vi "Draw.vi"(8 "error in (no error)":errorcluster, 10 "2D Picture in":picture, 11 "GrayScaleImage in":refnum<class "GrayScaleImage.lvclass">) -> (0 "error out":errorcluster, 2 "2D Picture out":picture, 3 "GrayScaleImage out":refnum<class "GrayScaleImage.lvclass">)   [LabVIEW 2021, in "Picture2D.lvlib" / "GrayScaleImage.lvclass"]
uses:
  GrayScaleImage.lvclass
  C:/GitHub/Picture2D/src/Picture/Image.lvclass
  ColorGrayScale/ColorGrayScale.lvclass
  Picture/Image.lvclass
  GrayScaleImage.lvclass/GrayScaleImage.ctl
  Picture2D/Picture2D.lvlib
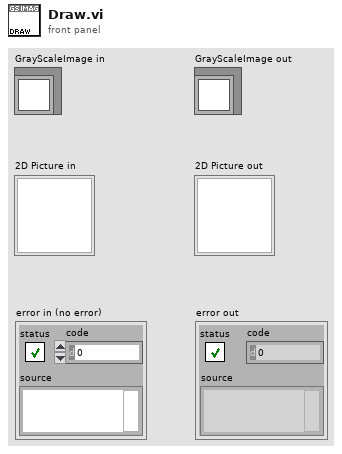
[diagram p1: front panel]
types:
  T1 = typedef "imagedata.ctl" = cluster{"image type":i32, "image depth":i32, "image":u8[], "mask":u8[], "colors":u32[], "Rectangle":cluster{"left":i16, "top":i16, "right":i16, "bottom":i16}}
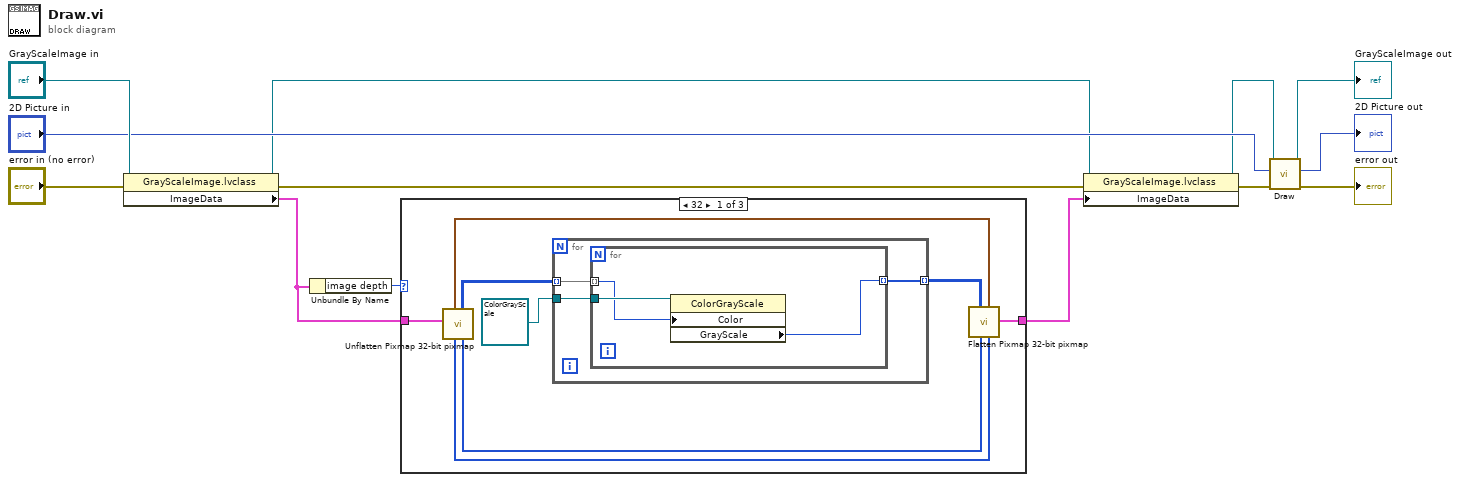
[diagram p0: block diagram]
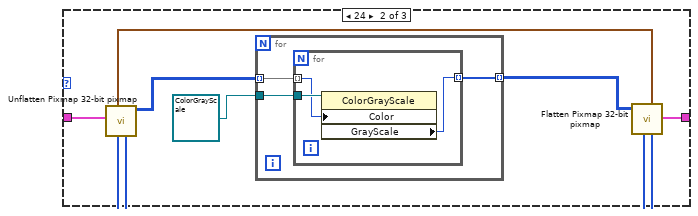
[diagram p2: hidden frame]
diagram:
  n1 = property class="GrayScaleImage.lvclass"(reference="GrayScaleImage in", error in="error in (no error)") -> (reference out=w2:refnum<class "GrayScaleImage.lvclass">, error out=w5:errorcluster, "ImageData"=w10:T1)
  n2 = Unbundle By Name(w10) -> ("image depth"=w13:i32)
  n3 = case shown="32" w13 {
    tunnel: w10 -> [w21 w35 w42]
    tunnel: [w20 w34 w42] -> w3
    frame 32 {
      n4 = call "Unflatten Pixmap 32-bit pixmap.vi"("image data"=w21) -> ("colors"=w17:u32[], "32-bit pixmap"=w15:u32[][], "mask"=w18:u8[], "top left"=w19:cluster{"x":i16, "y":i16})  [unwired: 3 in, 4 out]
      n5 = for {
        tunnel: refnum<class "ColorGrayScale.lvclass"> refnum ("ColorGrayScale") -> [w24]
        tunnel: [w23] -> w14 mode=indexing
        tunnel: w15 -> [w22] mode=indexing
        n6 = for {
          tunnel: w24 -> [w27]
          tunnel: [w25] -> w23 mode=indexing
          tunnel: w22 -> [w26] mode=indexing
          n7 = property class="ColorGrayScale"(reference=w27, "Color"=w26) -> ("GrayScale"=w25:u32)  [unwired: 1 in, 2 out]
        }
      }
      n8 = call "Flatten Pixmap 32-bit pixmap.vi"("mask"=w18, "top left"=w19, "colors"=w17, "32-bit pixmap"=w14) -> ("image data"=w20:T1)  [unwired: 7 in]
    }
    frame 24 {
      n9 = call "Unflatten Pixmap 32-bit pixmap.vi"("image data"=w35) -> ("24-bit pixmap"=w29:u32[][], "colors"=w31:u32[], "mask"=w32:u8[], "top left"=w33:cluster{"x":i16, "y":i16})  [unwired: 3 in, 4 out]
      n10 = for {
        tunnel: refnum<class "ColorGrayScale.lvclass"> refnum ("ColorGrayScale") -> [w38]
        tunnel: [w37] -> w28 mode=indexing
        tunnel: w29 -> [w36] mode=indexing
        n11 = for {
          tunnel: w38 -> [w41]
          tunnel: [w40] -> w37 mode=indexing
          tunnel: w36 -> [w39] mode=indexing
          n12 = property class="ColorGrayScale"(reference=w41, "Color"=w39) -> ("GrayScale"=w40:u32)  [unwired: 1 in, 2 out]
        }
      }
      n13 = call "Flatten Pixmap 32-bit pixmap.vi"("mask"=w32, "top left"=w33, "colors"=w31, "24-bit pixmap"=w28) -> ("image data"=w34:T1)  [unwired: 7 in]
    }
    frame Default {
    }
  }
  n14 = property class="GrayScaleImage.lvclass"(reference=w2, error in=w5, "ImageData"=w3) -> (reference out=w1:refnum<class "GrayScaleImage.lvclass">, error out=w4:errorcluster)
  n15 = call-parent "Draw.vi"("error in (no error)"=w4, "2D Picture in"="2D Picture in", "Picture in"=w1) -> ("error out"=→"error out":errorcluster, "2D Picture out"=→"2D Picture out":picture, "Picture out"=→"GrayScaleImage out":refnum<class "GrayScaleImage.lvclass">)  [unwired: 6 in]
